vi "PWM to Channel Settings.vi"(8 "error in":errorcluster, 9 "channel default values":dbl[](array[numeric]), 10 "channel names":string[](array[string]), 11 "SD Module in":refnum<class "SD Module.lvclass">) -> (0 "error out":errorcluster, 3 "channel settings":T1[](array[typedef]))   [LabVIEW 2017, in "Scan Engine Scripting.lvlib"]
uses:
  Scan Engine Scripting.lvlib
  Modules/Mode Classes/Controls/pwm channel settings.ctl
  Modules/Channel Classes/PWM Output Channel/Frequency.ctl
  Modules.lvlibp/SD Module/SD Module.lvclass
  Modules/Channel Classes/PWM Output Channel/PWM Output Channel.lvclass
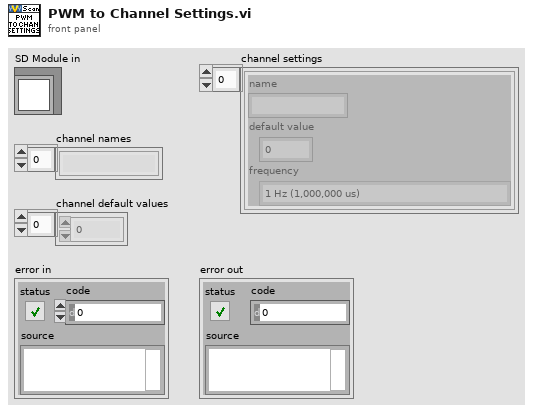
[diagram p1: front panel]
types:
  T1 = typedef "Scan Engine Scripting.lvlib/pwm channel settings.ctl" = cluster{"name":string, "default value":dbl, "frequency":T2}
  T2 = typedef "Scan Engine Scripting.lvlib/PWM Output Channel.lvclass/Frequency.ctl" = enum16{"1 Hz (1,000,000 us)", "50 Hz (20,000 us)", "250 Hz (4,000 us)", "500 Hz (2,000 us)", "1 kHz (1,000 us)", "5 kHz (200 us)", "10 kHz (100 us)", "20 kHz (50 us)"}
  T3 = typedef "Modules.lvlibp/SD Module.lvclass/PWM.ctl" = cluster{"PWM Channels":T4[]}
  T4 = typedef "Modules.lvlibp/SD Module.lvclass/PWM Channel.ctl" = cluster{"PWM frequency":u32}
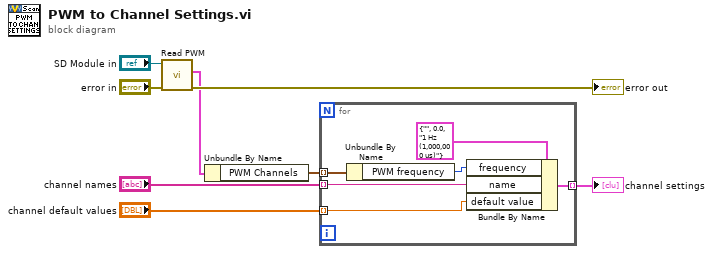
[diagram p0: block diagram]
diagram:
  n1 = call-dynamic "Read PWM.vi"("error in (no error)"="error in", "SD Module in"="SD Module in") -> ("error out"=→"error out":errorcluster, "PWM"=w3:T3)  [unwired: 7 in, 1 out]
  n2 = Unbundle By Name(w3) -> ("PWM Channels"=w4:T4[])
  n3 = for {
    tunnel: w4 -> [w14] mode=indexing
    tunnel: "channel names" -> [w11] mode=indexing
    tunnel: "channel default values" -> [w10] mode=indexing
    tunnel: [w9] -> w7 mode=indexing
    n4 = Unbundle By Name(w14) -> ("PWM frequency"=w12:u32)
    n5 = Bundle By Name(cluster=T1 {"name"="", "default value"=0.0, "frequency"=enum."1 Hz (1,000,000 us)"} ("channel settings"), "frequency"=w12, "name"=w11, "default value"=w10) -> (w9:T1)
  }
  "channel settings" <- w7
